vi "PH_Sound.Mai 2.vi"() -> (0 "... die Bäume schlagen aus.":cluster{"Tone":dbl, "Beats":i32}[](array[cluster]))   [LabVIEW 2009, in "PH_Sound.lvlib"]
doc: "\"... die Bäume schlagen aus.\""
uses:
  PH_Sound.lvlib
  PH_Common/PH_Audio/PH_3Oktaves.ctl
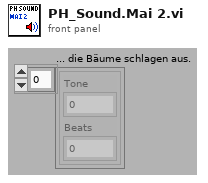
[diagram p1: front panel]
types:
  T1 = typedef "PH_3Oktaves.ctl" = dbl
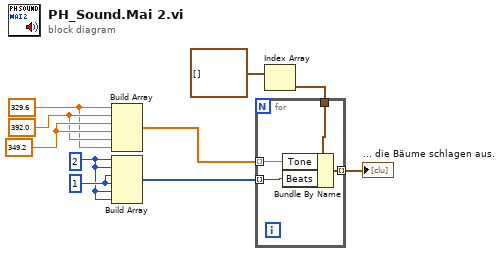
[diagram p0: block diagram]
diagram:
  w2 = 1 ("length")
  w1 = u32 2 ("y")
  w5 = T1 349.2 items=["c"=130.8, "cis"=138.6, "d"=146.8, "es"=155.6, "e"=164.8, "f"=174.6, "fis"=185.0, "g"=196.0, "as"=207.6, "a"=220.0, "b"=233.1, "h"=246.9, "c'"=261.6, "cis'"=277.2, "d'"=293.7, "es'"=311.1, "e'"=329.6, "f'"=349.2, "fis'"=370.0, "g'"=392.0, "as'"=415.3, "a'"=440.0, "b'"=466.2, "h'"=493.9, "c''"=523.3, "cis''"=554.4, "d''"=587.3, "es''"=622.3, "e''"=659.3, "f''"=689.5, "fis''"=740.0, "g''"=784.0, "as''"=830.6, "a''"=880.0, "b''"=932.3, "h''"=987.8, "c'''"=1047.0] ("3 Octaves")
  w4 = T1 392.0 items=["c"=130.8, "cis"=138.6, "d"=146.8, "es"=155.6, "e"=164.8, "f"=174.6, "fis"=185.0, "g"=196.0, "as"=207.6, "a"=220.0, "b"=233.1, "h"=246.9, "c'"=261.6, "cis'"=277.2, "d'"=293.7, "es'"=311.1, "e'"=329.6, "f'"=349.2, "fis'"=370.0, "g'"=392.0, "as'"=415.3, "a'"=440.0, "b'"=466.2, "h'"=493.9, "c''"=523.3, "cis''"=554.4, "d''"=587.3, "es''"=622.3, "e''"=659.3, "f''"=689.5, "fis''"=740.0, "g''"=784.0, "as''"=830.6, "a''"=880.0, "b''"=932.3, "h''"=987.8, "c'''"=1047.0] ("3 Octaves")
  w3 = T1 329.6 items=["c"=130.8, "cis"=138.6, "d"=146.8, "es"=155.6, "e"=164.8, "f"=174.6, "fis"=185.0, "g"=196.0, "as"=207.6, "a"=220.0, "b"=233.1, "h"=246.9, "c'"=261.6, "cis'"=277.2, "d'"=293.7, "es'"=311.1, "e'"=329.6, "f'"=349.2, "fis'"=370.0, "g'"=392.0, "as'"=415.3, "a'"=440.0, "b'"=466.2, "h'"=493.9, "c''"=523.3, "cis''"=554.4, "d''"=587.3, "es''"=622.3, "e''"=659.3, "f''"=689.5, "fis''"=740.0, "g''"=784.0, "as''"=830.6, "a''"=880.0, "b''"=932.3, "h''"=987.8, "c'''"=1047.0] ("3 Octaves")
  n1 = Build Array(w3, w4, w5, w5, w4, w3) -> (w9:T1[])
  n2 = Build Array(w1, w1, w2, w2, w1, w1) -> (w8:u32[])
  n3 = Index Array(array=cluster{"Tone":dbl, "Beats":i32}[] [] ("Song")) -> (element=w6:cluster{"Tone":dbl, "Beats":i32})  [unwired: 1 in]
  n4 = for {
    tunnel: w9 -> [w13] mode=indexing
    tunnel: w6 -> [w14]
    tunnel: [w12] -> w10 mode=indexing
    tunnel: w8 -> [w11] mode=indexing
    n5 = Bundle By Name(cluster=w14, "Tone"=w13, "Beats"=w11) -> (w12:cluster{"Tone":dbl, "Beats":i32})
  }
  "... die Bäume schlagen aus." <- w10
